vi "Perform Action.vi"(8 "error in":errorcluster, 10 "Input":variant, 11 "AO DAQmx DC CFG in":refnum<class "AO DAQmx DC CFG.lvclass">) -> (0 "error out":errorcluster, 2 "Output":variant, 3 "AO DAQmx DC CFG out":refnum<class "AO DAQmx DC CFG.lvclass">)   [LabVIEW 2023, in "AO DAQmx DC CFG.lvclass"]
uses:
  AO DAQmx DC CFG.lvclass
  Configuration/Configuration Semaphore/CFG Semaphore.lvclass
  DAQmx/DAQmx Base CFG/DAQmx Base CFG.lvclass
  <vilib>/DAQmx/write.llb/DAQmx Write (Analog 1D DBL NChan 1Samp).vi
  DAQmx/BufferWrites1SamDBL/BufferWrites1SamDBL.lvclass
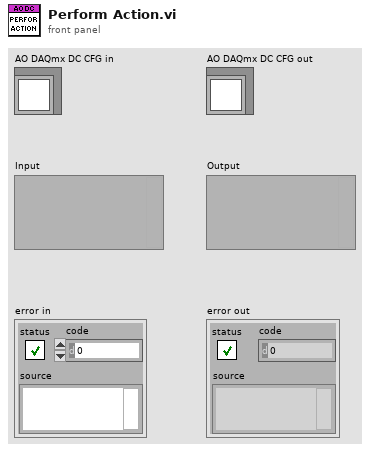
[diagram p1: front panel]
types:
  T1 = typedef "Semaphore RefNum" = refnum<k1>
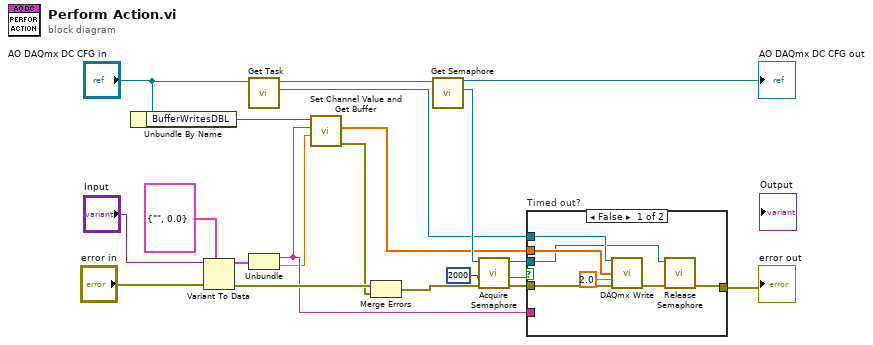
[diagram p0: block diagram]
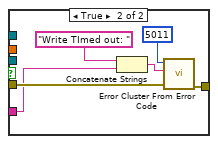
[diagram p2: hidden frame]
diagram:
  n1 = Unbundle By Name("AO DAQmx DC CFG in") -> ("BufferWritesDBL"=w17:refnum<class "BufferWrites1SamDBL.lvclass">)
  n2 = Variant To Data(error in="error in", type=cluster{"Channel":string, "Level":dbl} {"Channel"="", "Level"=0.0}, Variant="Input") -> (data=w16:cluster{"Channel":string, "Level":dbl}, error out=w18:errorcluster)
  n3 = call "Get Task.vi"("DAQmx Base CFG in"="AO DAQmx DC CFG in") -> ("Task"=w3:refnum<k21>, "DAQmx Base CFG out"=w9:refnum<class "AO DAQmx DC CFG.lvclass">)  [unwired: 9 in]
  n4 = Unbundle(w16) -> ("Channel"=w2:string, "Level"=w1:dbl)
  n5 = call-dynamic "Set Channel Value and Get Buffer.vi"("Value"=w1, "Channel"=w2, "BufferWritesDBL in"=w17) -> ("error out"=w4:errorcluster, "Write Buffer"=w10:dbl[])  [unwired: 6 in, 1 out]
  n6 = Merge Errors(w18, w4) -> (w5:errorcluster)
  n7 = call "Get Semaphore.vi"("CFG Base in"=w9) -> ("Semaphore"=w13:T1, "CFG Base out"=→"AO DAQmx DC CFG out":refnum<class "AO DAQmx DC CFG.lvclass">)  [unwired: 9 in]
  n8 = call <vilib>:"Acquire Semaphore.vi"("error in (no error)"=w5, "ms timeout (-1)"=2000, "semaphore"=w13) -> ("error out"=w14:errorcluster, "timed out"=w12:bool, "semaphore out"=w6:T1)  [unwired: 2 in]
  n9 = case "Timed out?" shown="False" w12 {
    tunnel: w14 -> [w28 w33]
    tunnel: w10 -> [w27 _]
    tunnel: w3 -> [w25 _]
    tunnel: [w23 w34] -> w8
    tunnel: w2 -> [_ w29]
    tunnel: w6 -> [w22 _]
    frame False {
      n10 = call-poly <vilib>:"DAQmx Write.vi"("task/channels in"=w25, "data"=w27, "timeout"=2.0, "error in"=w28) -> ("error out"=w24:errorcluster)  [unwired: 9 in, 2 out]
      n11 = call <vilib>:"Release Semaphore.vi"("error in (no error)"=w24, "semaphore"=w22) -> ("error out"=w23:errorcluster)  [unwired: 4 in, 1 out]
    }
    frame True {
      n12 = Concatenate Strings("Write TImed out: " ("string"), w29) -> (w31:string)
      n13 = call <vilib>:"Error Cluster From Error Code.vi"("error in (no error)"=w33, "error message (\"\")"=w31, "error code (0)"=5011) -> ("error out"=w34:errorcluster)  [unwired: 6 in]
    }
  }
  "error out" <- w8
